vi "CS_Contents_User.vi"   [LabVIEW 2014]
doc: "This \"contents\" VI contains all components of CS, which are specific for YOU, a CS user. Add your own stuff here."
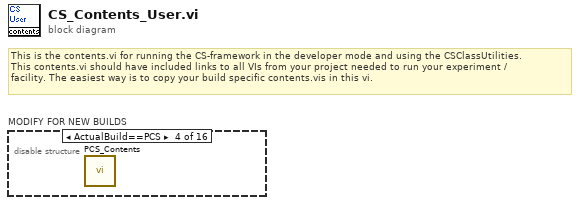
[diagram p0: block diagram]
diagram:
  # "This is the contents.vi for running the CS-framework in the developer mode and using the CSClassUtilities.\nThis contents.vi should have included links to all VIs from your project needed to run your experiment / \nfacility. The easiest way is to copy your build specific contents.vis in this vi."
  n1 = disable-structure "MODIFY FOR NEW BUILDS" shown="ActualBuild==PCS" {
    frame condition #0 {
    }
    frame condition #1 {
    }
    frame condition #2 {
    }
    frame condition #3 (active) {
      n2 = call "PCS_Contents.vi"() -> ()  [unwired: 1 in]
    }
    frame condition #4 {
    }
    frame condition #5 {
    }
    frame condition #6 {
    }
    frame condition #7 {
    }
    frame condition #8 {
    }
    frame condition #9 {
    }
    frame condition #10 {
    }
    frame condition #11 {
    }
    frame condition #12 {
    }
    frame condition #13 {
    }
    frame condition #14 {
    }
    frame condition #15 {
    }
  }
